vi "Close File.vi"(8 "error in":errorcluster, 11 "refnum":refnum<file>) -> (0 "error out":errorcluster)   [LabVIEW 2023]
doc: "Closes a file.\n\nUse this VI as a the teardown VI Write to File.lvtest and Read from File.lvtest"
panel:
  # "Overview: Use this VI as the teardown VI for Write to File.lvtest and Read from File.lvtest.\nRequirements: LabVIEW Full Development System, Unit Test Framework Toolkit\nInstructions: \n1.  In the Project Explorer window, double-click Write to File.lvtest or Read from File.lvtest to display the Test Properties dialog box.\n2.  Select Setup/Teardown from the Category list to display the Setup/Teardown page. You can understand how LabVIEW passes values among the setup VI, the VI under test, and the teardown VI. LabVIEW compares the outputs of the teardown VI with the expected values."
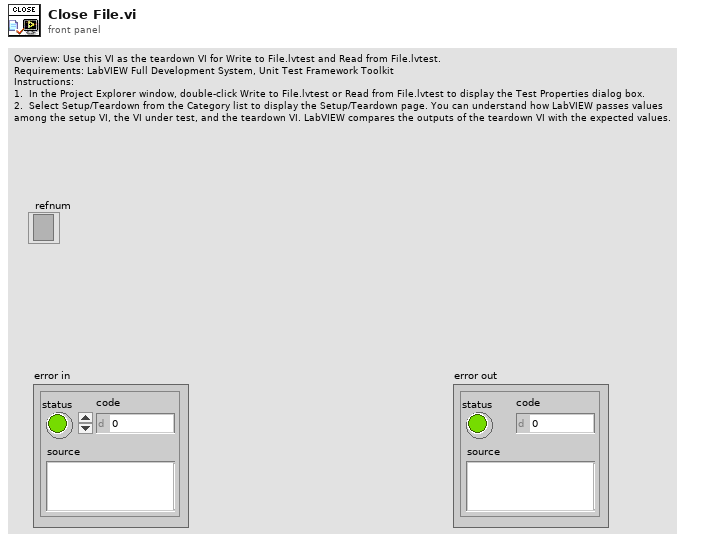
[diagram p1: front panel]
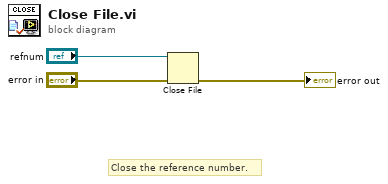
[diagram p0: block diagram]
diagram:
  # "Close the reference number."
  n1 = Close File(refnum="refnum", error in="error in") -> (error out=→"error out":errorcluster)  [unwired: 1 out]
